vi "List Dependencies Recursive.vi"(8 "error in (no error)":errorcluster, 11 "SMOs in":refnum<class "SMO.lvclass">[](array[class])) -> (0 "error out":errorcluster, 1 "Names":string[](array[string]), 2 "[Dependencies]":refnum<class "SMO.lvclass">[](array[class]), 3 "SMOs out":refnum<class "SMO.lvclass">[](array[class]))   [LabVIEW 2019, in "Logger.Error.lvlib" / "Logger.Error.lvclass"]
uses:
  Logger.Error.lvclass
  <vilib>/JKI/JKI SMO/SMO/SMO.lvclass
  <vilib>/JKI/JKI SMO/SMO/SMO.lvclass/SMO.ctl
  <vilib>/JKI/JKI SMO/SMO/Private/GetDependencies.vi
  <vilib>/JKI/JKI SMO/Support/Attribute.Dependencies/List Dependencies.vi
  <vilib>/JKI/JKI SMO/SMO/Private/GetVariant(Attr).vi
  <vilib>/JKI/JKI SMO/SMO/Private/ReftoDVR--SMO.vi
  <vilib>/JKI/JKI SMO/Support/Attribute.Dependencies/Get GUIDs.vi
  <vilib>/JKI/JKI SMO/SMO/isStateMachineObject.vi
  <vilib>/JKI/JKI SMO/Support/Attribute.Dependencies/Attribute.Dependencies.lvclass
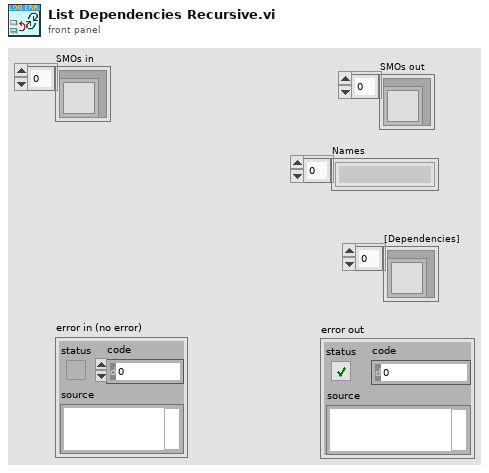
[diagram p1: front panel]
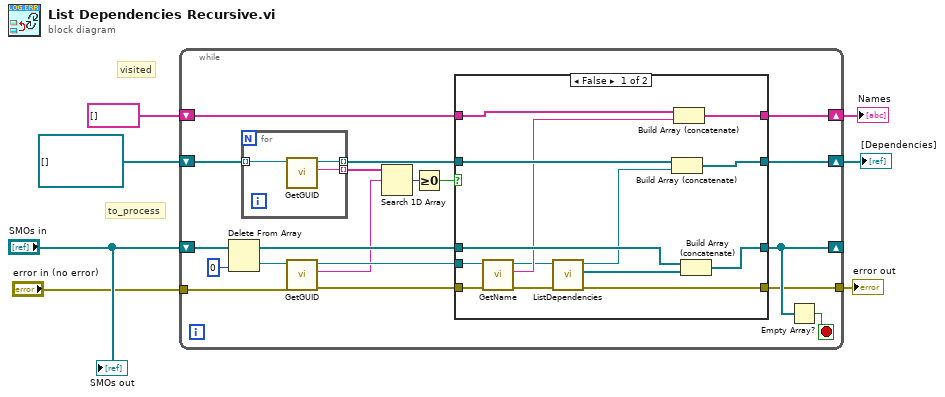
[diagram p0: block diagram]
diagram:
  # "visited"
  # "to_process"
  n1 = while {
    shift-right: [w20] -> _
    shift-left: "SMOs in" -> [w26]
    shift-right: [w22] -> w6
    shift-left: refnum<class "SMO.lvclass">[] [] ("Visited") -> [w16]
    shift-right: [w18] -> w4
    shift-left: string[] [] -> [w17]
    tunnel: "error in (no error)" -> [w10]
    tunnel: [w8] -> w1
    stop <- w19 stop-if-true
    n2 = Delete From Array(array=w26, index=0) -> (deleted portion=w13:refnum<class "SMO.lvclass">, array with subset deleted=w21:refnum<class "SMO.lvclass">[])  [unwired: 1 in]
    n3 = for {
      tunnel: w16 -> [w29] mode=indexing
      tunnel: [w28] -> w15 mode=indexing
      tunnel: [w27] -> w14 mode=indexing
      n4 = call <vilib>:"GetGUID.vi"("SMO"=w29) -> ("GUID"=w27:string, "SMO out"=w28:refnum<class "SMO.lvclass">)  [unwired: 8 in, 1 out]
    }
    n5 = call <vilib>:"GetGUID.vi"("error in (no error)"=w10, "SMO"=w13) -> ("error out"=w9:errorcluster, "GUID"=w11:string, "SMO out"=w12:refnum<class "SMO.lvclass">)  [unwired: 7 in]
    n6 = Search 1D Array(1D array=w14, element=w11) -> (index of element=w24:i32)  [unwired: 1 in]
    n7 = Greater Or Equal To 0?(x=w24) -> (x >= 0?=w25:bool)
    n8 = case shown="False" w25 {
      tunnel: w12 -> [w35 _]
      tunnel: [w42 w47] -> w22
      tunnel: w15 -> [w43 w47]
      tunnel: [w40 w46] -> w20
      tunnel: w21 -> [w39 w46]
      tunnel: [w37 w45] -> w18
      tunnel: w17 -> [w36 w45]
      tunnel: w9 -> [w32 w44]
      tunnel: [w30 w44] -> w8
      frame False {
        n9 = call <vilib>:"GetName.vi"("error in (no error)"=w32, "SMO"=w35) -> ("error out"=w31:errorcluster, "Name"=w34:string, "SMO out"=w33:refnum<class "SMO.lvclass">)  [unwired: 6 in, 1 out]
        n10 = call <vilib>:"ListDependencies.vi"("error in (no error)"=w31, "SMO in"=w33) -> ("error out"=w30:errorcluster, "[Dependencies]"=w41:refnum<class "SMO.lvclass">[], "SMO out"=w38:refnum<class "SMO.lvclass">)  [unwired: 6 in, 1 out]
        n11 = Build Array (concatenate)(w43, w38) -> (w42:refnum<class "SMO.lvclass">[])
        n12 = Build Array (concatenate)(w36, w34) -> (w37:string[])
        n13 = Build Array (concatenate)(w39, w41) -> (w40:refnum<class "SMO.lvclass">[])
      }
      frame True {
      }
    }
    n14 = Empty Array?(array=w20) -> (empty?=w19:bool)
  }
  "[Dependencies]" <- w6
  "Names" <- w4
  "error out" <- w1
  "SMOs out" <- "SMOs in"
